vi "SmartMotor_SendCommands-MultipleMotors.vi"(6 "ReadWait":u32=50, 8 "error in (no error)":errorcluster, 9 "MotorSpecifier(None) in":T1, 10 "MotorStartupCmds":string[](array[string]), 11 "VISA Refnum in":refnum<visa-resource-name>) -> (0 "error out":errorcluster, 1 "cmd str out":string[](array[string]), 3 "VISA Refnum out":refnum<visa-resource-name>)   [LabVIEW 2020]
doc: "Developed by Kevin Thompson\nkevin@thompsonengineering.net\n\nCopyright 2018-2020\nThompson Engineering, LLC"
uses:
  TD SerialBusMotorSpecifier_enum.ctl
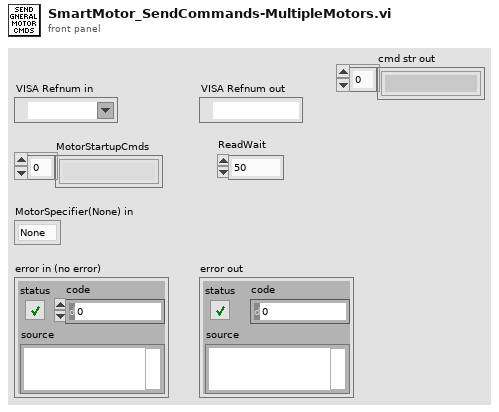
[diagram p1: front panel]
types:
  T1 = typedef "TD SerialBusMotorSpecifier_enum.ctl" = enum16{"None", "Global", "M1", "M2", "M3"}
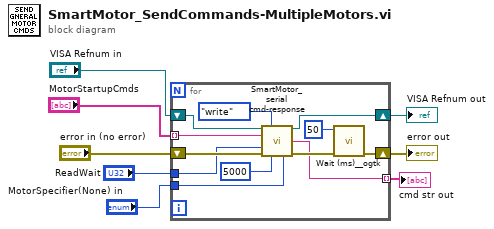
[diagram p0: block diagram]
diagram:
  n1 = for {
    shift-right: [w18] -> w7
    shift-left: "VISA Refnum in" -> [w19]
    tunnel: "MotorStartupCmds" -> [w17] mode=indexing
    shift-right: [w13] -> w8
    shift-left: "error in (no error)" -> [w16]
    tunnel: "MotorSpecifier(None) in" -> [w11]
    tunnel: [w10] -> w2 mode=indexing
    tunnel: "ReadWait" -> [w9]
    n2 = call "SmartMotor_serial cmd-response.vi"("VISA In"=w19, "mode"=enum16{"wr & rd", "write", "read"}."write", "cmd"=w17, "ReadWait"=w9, "error in"=w16, "Sem Timeout (5000)"=5000, "MotorSpecifier(None)"=w11) -> ("VISA out"=w18:refnum<visa-resource-name>, "cmd str out"=w10:string, "error out"=w14:errorcluster)  [unwired: 4 in, 2 out]
    n3 = call <userlib>:"Wait (ms)__ogtk.vi"("error in (no error)"=w14, "milliseconds to wait"=u32 50) -> ("error out"=w13:errorcluster)  [unwired: 8 in, 1 out]
  }
  "error out" <- w8
  "VISA Refnum out" <- w7
  "cmd str out" <- w2
